vi "TranslateObjects.vi"(8 "errorIN":errorcluster, 10 "Cle":string, 11 "AllObjs[]In":refnum<vi>[](array[refnum])) -> (0 "error out":errorcluster, 3 "AllObjs[]Out":refnum<vi>[](array[refnum]))   [LabVIEW 2013]
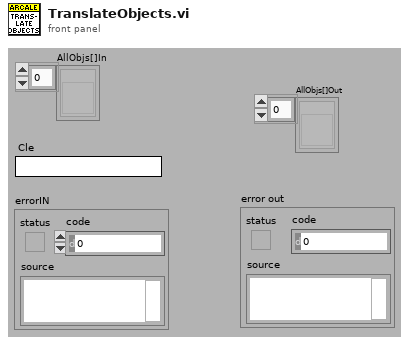
[diagram p1: front panel]
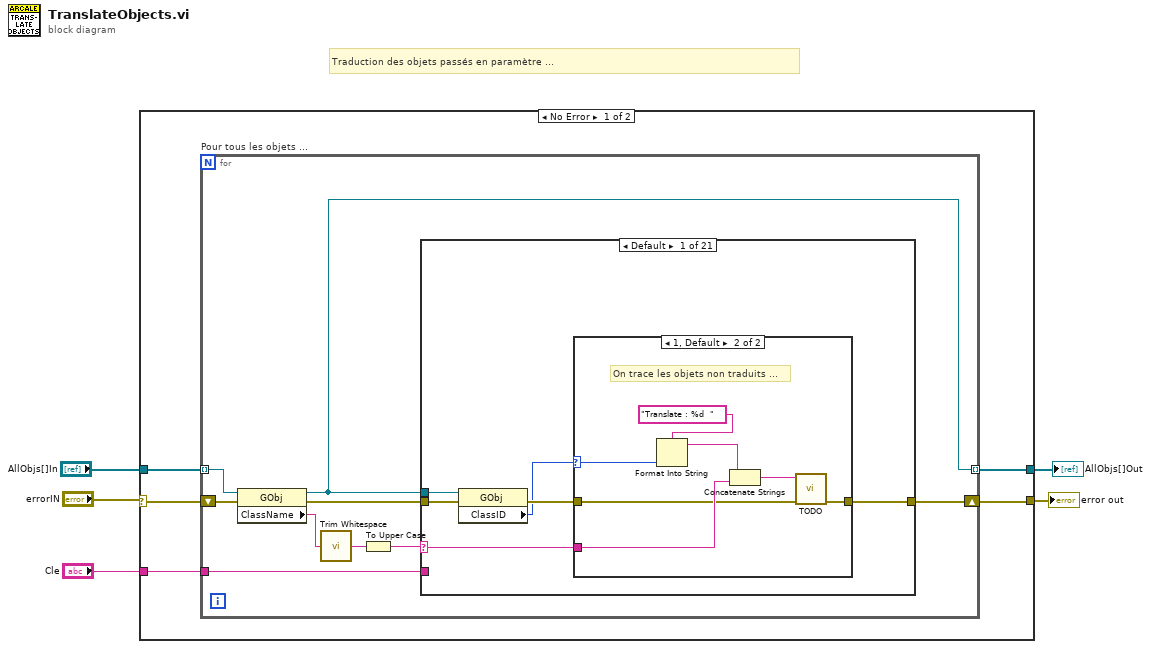
[diagram p0: block diagram]
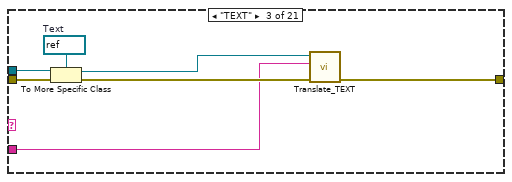
[diagram p4: hidden frame]
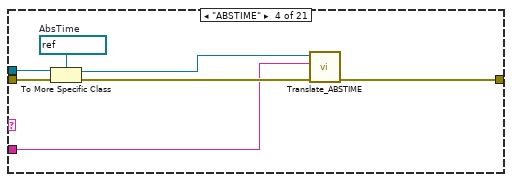
[diagram p5: hidden frame]
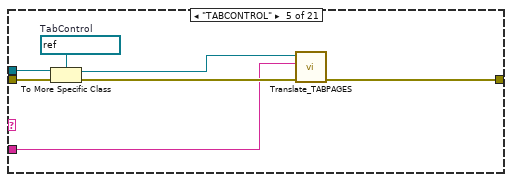
[diagram p6: hidden frame]
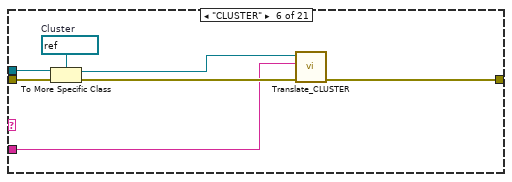
[diagram p7: hidden frame]
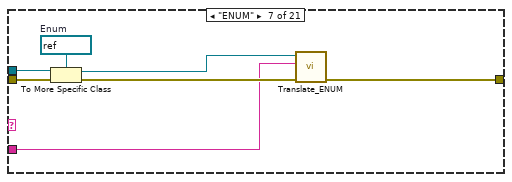
[diagram p8: hidden frame]
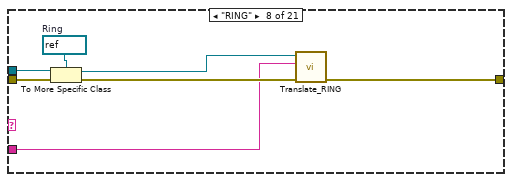
[diagram p9: hidden frame]
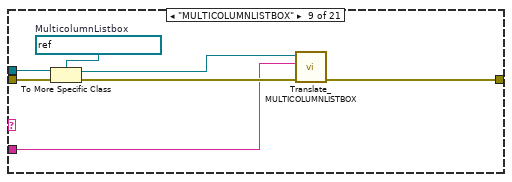
[diagram p10: hidden frame]
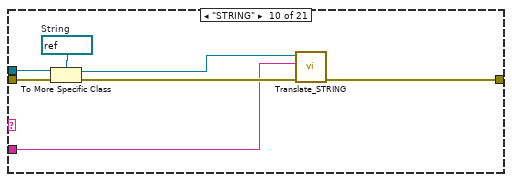
[diagram p11: hidden frame]
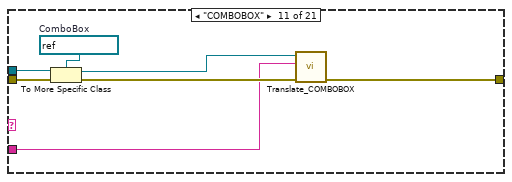
[diagram p12: hidden frame]
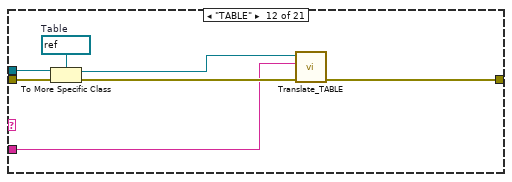
[diagram p13: hidden frame]
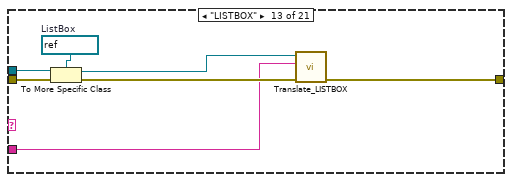
[diagram p14: hidden frame]
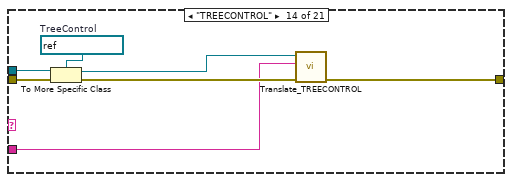
[diagram p15: hidden frame]
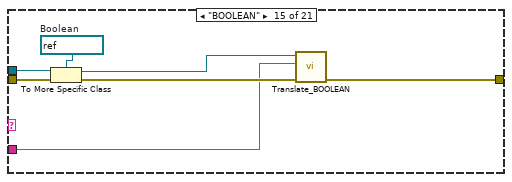
[diagram p16: hidden frame]
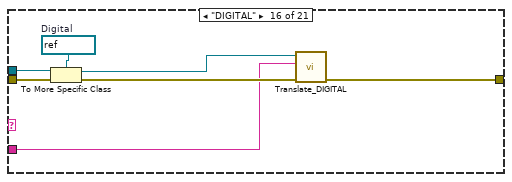
[diagram p17: hidden frame]
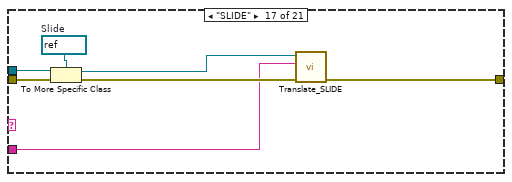
[diagram p18: hidden frame]
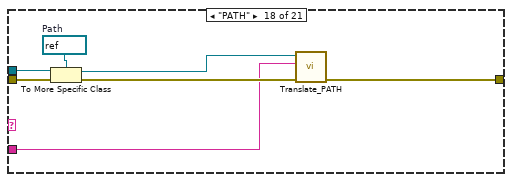
[diagram p19: hidden frame]
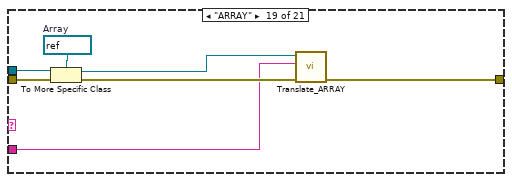
[diagram p20: hidden frame]
diagram:
  # "Traduction des objets passés en paramètre ..."
  n1 = case shown="No Error" "errorIN" {
    selector: "errorIN" -> [w9 w169]
    tunnel: [w6 w169] -> w4
    tunnel: "AllObjs[]In" -> [w10 w168]
    tunnel: [w7 w168] -> w2
    tunnel: "Cle" -> [w8 _]
    frame No Error {
      n2 = for "Pour tous les objets ..." {
        tunnel: w10 -> [w19] mode=indexing
        shift-right: [w15] -> w6
        shift-left: w9 -> [w18]
        tunnel: w8 -> [w13]
        tunnel: [w14] -> w7 mode=indexing
        n3 = property class="GObj"(reference=w19, error in=w18) -> (reference out=w14:refnum<vi>, error out=w11:errorcluster, "ClassName"=w17:string)
        n4 = call <vilib>:"Trim Whitespace.vi"("string"=w17) -> ("trimmed string"=w16:string)  [unwired: 1 in]
        n5 = To Upper Case(1:w16) -> (0:w12:string)
        n6 = case shown="Default" w12 {
          selector: w12 -> [w24 _ _ _ _ _ _ _ _ _ _ _ _ _ _ _ _ _ _ _ _]
          tunnel: w11 -> [w23 w34 w40 w47 w54 w61 w68 w75 w82 w89 w96 w103 w110 w117 w124 w131 w138 w145 w152 w159 w166]
          tunnel: [w25 w34 w36 w43 w49 w56 w63 w70 w77 w84 w91 w98 w105 w112 w119 w126 w133 w140 w148 w154 w161] -> w15
          tunnel: w14 -> [w21 _ w41 w48 w55 w62 w69 w76 w83 w90 w97 w104 w111 w118 w125 w132 w139 w146 w153 w160 w167]
          tunnel: w13 -> [_ _ w37 w44 w51 w58 w65 w72 w79 w86 w93 w100 w107 w114 w121 w128 w135 w142 w149 w156 w163]
          frame Default {
            n7 = property class="GObj"(reference=w21, error in=w23) -> (error out=w22:errorcluster, "ClassID"=w20:u32)  [unwired: 1 out]
            n8 = case shown="1, Default" w20 {
              selector: w20 -> [_ w27]
              tunnel: [w26 w33] -> w25
              tunnel: w24 -> [_ w32]
              tunnel: w22 -> [w26 w30]
              frame 6 {
                # "6 : XControl"
              }
              frame 1, Default {
                # "On trace les objets non traduits ..."
                n9 = Format Into String(format string="Translate : %d  " ("string"), w27) -> (resulting string=w28:string)  [unwired: 2 in, 1 out]
                n10 = Concatenate Strings(w28, w32) -> (w31:string)
                n11 = call "TODO.vi"("error in (no error)"=w30, "Message"=w31) -> ("error out"=w33:errorcluster)  [unwired: 9 in]
              }
            }
          }
          frame "DECORATION", "PICTURE", "SUBPANEL", "VIREFNUM" {
            # "Non traduits ..."
          }
          frame "TEXT" {
            w39 = refnum<vi> refnum  # Text
            n12 = To More Specific Class(target class=w39, reference=w41, error in=w40) -> (specific class reference=w35:refnum<vi>, error out=w38:errorcluster)
            n13 = call "Translate_TEXT.vi"("error In"=w38, "Cle"=w37, "Txt Refnum"=w35) -> ("error out"=w36:errorcluster)  [unwired: 8 in]
          }
          frame "ABSTIME" {
            w46 = refnum<vi> refnum  # AbsTime
            n14 = To More Specific Class(target class=w46, reference=w48, error in=w47) -> (specific class reference=w42:refnum<vi>, error out=w45:errorcluster)
            n15 = call "Translate_ABSTIME.vi"("error In"=w45, "Cle"=w44, "AbsTime Refnum"=w42) -> ("error out"=w43:errorcluster)  [unwired: 8 in]
          }
          frame "TABCONTROL" {
            w53 = refnum<vi> refnum  # TabControl
            n16 = To More Specific Class(target class=w53, reference=w55, error in=w54) -> (specific class reference=w50:refnum<vi>, error out=w52:errorcluster)
            n17 = call "Translate_TABPAGES.vi"("error IN"=w52, "Cle"=w51, "TabCtl Refnum"=w50) -> ("error out"=w49:errorcluster)  [unwired: 8 in]
          }
          frame "CLUSTER" {
            w60 = refnum<vi> refnum  # Cluster
            n18 = To More Specific Class(target class=w60, reference=w62, error in=w61) -> (specific class reference=w57:refnum<vi>, error out=w59:errorcluster)
            n19 = call "Translate_CLUSTER.vi"("error IN"=w59, "Cle"=w58, "Clust Refnum"=w57) -> ("error out"=w56:errorcluster)  [unwired: 8 in]
          }
          frame "ENUM" {
            w67 = refnum<vi> refnum  # Enum
            n20 = To More Specific Class(target class=w67, reference=w69, error in=w68) -> (specific class reference=w64:refnum<vi>, error out=w66:errorcluster)
            n21 = call "Translate_ENUM.vi"("error IN"=w66, "Cle"=w65, "Enum Refnum"=w64) -> ("error out"=w63:errorcluster)  [unwired: 8 in]
          }
          frame "RING" {
            w74 = refnum<vi> refnum  # Ring
            n22 = To More Specific Class(target class=w74, reference=w76, error in=w75) -> (specific class reference=w71:refnum<vi>, error out=w73:errorcluster)
            n23 = call "Translate_RING.vi"("error IN"=w73, "Cle"=w72, "Ring Refnum"=w71) -> ("error out"=w70:errorcluster)  [unwired: 8 in]
          }
          frame "MULTICOLUMNLISTBOX" {
            w81 = refnum<vi> refnum  # MulticolumnListbox
            n24 = To More Specific Class(target class=w81, reference=w83, error in=w82) -> (specific class reference=w78:refnum<vi>, error out=w80:errorcluster)
            n25 = call "Translate_MULTICOLUMNLISTBOX.vi"("error IN"=w80, "Cle"=w79, "MCListbox Refnum"=w78) -> ("error out"=w77:errorcluster)  [unwired: 8 in]
          }
          frame "STRING" {
            w88 = refnum<vi> refnum  # String
            n26 = To More Specific Class(target class=w88, reference=w90, error in=w89) -> (specific class reference=w85:refnum<vi>, error out=w87:errorcluster)
            n27 = call "Translate_STRING.vi"("error IN"=w87, "Cle"=w86, "Str Refnum"=w85) -> ("error out"=w84:errorcluster)  [unwired: 8 in]
          }
          frame "COMBOBOX" {
            w95 = refnum<vi> refnum  # ComboBox
            n28 = To More Specific Class(target class=w95, reference=w97, error in=w96) -> (specific class reference=w92:refnum<vi>, error out=w94:errorcluster)
            n29 = call "Translate_COMBOBOX.vi"("error IN"=w94, "Cle"=w93, "CmbBox Refnum"=w92) -> ("error out"=w91:errorcluster)  [unwired: 8 in]
          }
          frame "TABLE" {
            w102 = refnum<vi> refnum  # Table
            n30 = To More Specific Class(target class=w102, reference=w104, error in=w103) -> (specific class reference=w99:refnum<vi>, error out=w101:errorcluster)
            n31 = call "Translate_TABLE.vi"("error IN"=w101, "Cle"=w100, "Tbl Refnum"=w99) -> ("error out"=w98:errorcluster)  [unwired: 8 in]
          }
          frame "LISTBOX" {
            w109 = refnum<vi> refnum  # ListBox
            n32 = To More Specific Class(target class=w109, reference=w111, error in=w110) -> (specific class reference=w106:refnum<vi>, error out=w108:errorcluster)
            n33 = call "Translate_LISTBOX.vi"("error IN"=w108, "Cle"=w107, "LstBox Refnum"=w106) -> ("error out"=w105:errorcluster)  [unwired: 8 in]
          }
          frame "TREECONTROL" {
            w116 = refnum<vi> refnum  # TreeControl
            n34 = To More Specific Class(target class=w116, reference=w118, error in=w117) -> (specific class reference=w113:refnum<vi>, error out=w115:errorcluster)
            n35 = call "Translate_TREECONTROL.vi"("error IN"=w115, "Cle"=w114, "Tree Refnum"=w113) -> ("error out"=w112:errorcluster)  [unwired: 8 in]
          }
          frame "BOOLEAN" {
            w123 = refnum<vi> refnum  # Boolean
            n36 = To More Specific Class(target class=w123, reference=w125, error in=w124) -> (specific class reference=w120:refnum<vi>, error out=w122:errorcluster)
            n37 = call "Translate_BOOLEAN.vi"("error IN"=w122, "Cle"=w121, "Bool Refnum"=w120) -> ("error out"=w119:errorcluster)  [unwired: 8 in]
          }
          frame "DIGITAL" {
            w130 = refnum<vi> refnum  # Digital
            n38 = To More Specific Class(target class=w130, reference=w132, error in=w131) -> (specific class reference=w127:refnum<vi>, error out=w129:errorcluster)
            n39 = call "Translate_DIGITAL.vi"("error IN"=w129, "Cle"=w128, "DigNum Refnum"=w127) -> ("error out"=w126:errorcluster)  [unwired: 8 in]
          }
          frame "SLIDE" {
            w137 = refnum<vi> refnum  # Slide
            n40 = To More Specific Class(target class=w137, reference=w139, error in=w138) -> (specific class reference=w134:refnum<vi>, error out=w136:errorcluster)
            n41 = call "Translate_SLIDE.vi"("error IN"=w136, "Cle"=w135, "Slide Refnum"=w134) -> ("error out"=w133:errorcluster)  [unwired: 8 in]
          }
          frame "PATH" {
            w144 = refnum<vi> refnum  # Path
            n42 = To More Specific Class(target class=w144, reference=w146, error in=w145) -> (specific class reference=w141:refnum<vi>, error out=w143:errorcluster)
            n43 = call "Translate_PATH.vi"("error IN"=w143, "Cle"=w142, "Path Refnum"=w141) -> ("error out"=w140:errorcluster)  [unwired: 8 in]
          }
          frame "ARRAY" {
            w151 = refnum<vi> refnum  # Array
            n44 = To More Specific Class(target class=w151, reference=w153, error in=w152) -> (specific class reference=w147:refnum<vi>, error out=w150:errorcluster)
            n45 = call "Translate_ARRAY.vi"("error IN"=w150, "Cle"=w149, "Arr Refnum"=w147) -> ("error out"=w148:errorcluster)  [unwired: 8 in]
          }
          frame "XYGRAPH" {
            w158 = refnum<vi> refnum  # XYGraph
            n46 = To More Specific Class(target class=w158, reference=w160, error in=w159) -> (specific class reference=w155:refnum<vi>, error out=w157:errorcluster)
            n47 = call "Translate_XYGRAPH.vi"("error IN"=w157, "Cle"=w156, "XYRefnum"=w155) -> ("error out"=w154:errorcluster)  [unwired: 8 in]
          }
          frame "ACTIVEXCONTAINER" {
            w165 = refnum<vi> refnum  # ActiveXContainer
            n48 = To More Specific Class(target class=w165, reference=w167, error in=w166) -> (specific class reference=w162:refnum<vi>, error out=w164:errorcluster)
            n49 = call "Translate_ACTIVXCONTAINER.vi"("error IN"=w164, "Cle"=w163, "XYRefnum"=w162) -> ("error out"=w161:errorcluster)  [unwired: 8 in]
          }
        }
      }
    }
    frame Error {
    }
  }
  "error out" <- w4
  "AllObjs[]Out" <- w2
